vi "Append Text to Rich Text Box.vi"(8 "error in (no error)":errorcluster, 9 "Text Formatting":T1={"Font"="", "Text Color"=enum."Unchanged", "Background Color"=enum."Unchanged", "Style"=enum."Regular", "Font Size"=-1.0, "Alignment"=enum."Left"} {"Font Size" min=6.0 step=1.0}, 10 "String":string="\r\nALiX stopped on 7/2/2016 at 12:14 PM\n\r\n", 11 ".NET Refnum in":refnum<k24>) -> (0 "Error Out":errorcluster, 2 "Rtf Content":string, 3 ".NET Refnum out":refnum<k24>)   [LabVIEW 2021, in "Rich Text Box.lvlib"]
uses:
  Rich Text Box.lvlib
  System.Windows.Forms
  Text Formatting.ctl
  Text Colors.ctl
  Text Style.ctl
  Text Alignment.ctl
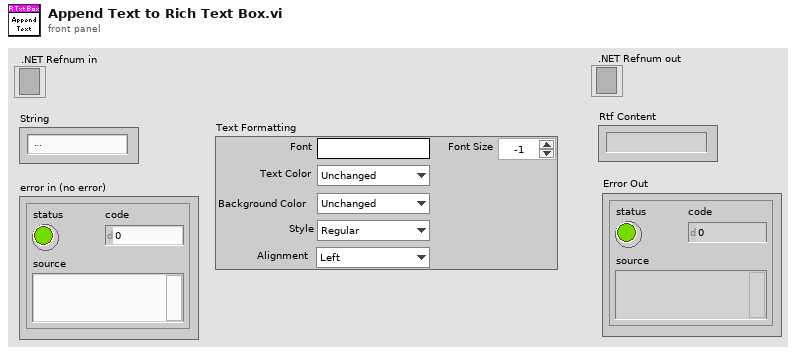
[diagram p1: front panel]
types:
  T1 = typedef "Rich Text Box.lvlib/Text Formatting.ctl" = cluster{"Font":string, "Text Color":T2, "Background Color":T2, "Style":T3, "Font Size":dbl, "Alignment":T4}
  T2 = typedef "Rich Text Box.lvlib/Text Colors.ctl" = enum16{"Unchanged", "Black", "Blue", "Cyan", "Maroon", "Gray", "Violet", "Green", "Light Green", "Orange", "Yellow", "Magenta", "Red", "White"}
  T3 = typedef "Rich Text Box.lvlib/Text Style.ctl" = enum16{"Regular", "Bold", "Italic", "Underline", "Strikeout"}
  T4 = typedef "Rich Text Box.lvlib/Text Alignment.ctl" = enum16{"Left", "Right", "Center"}
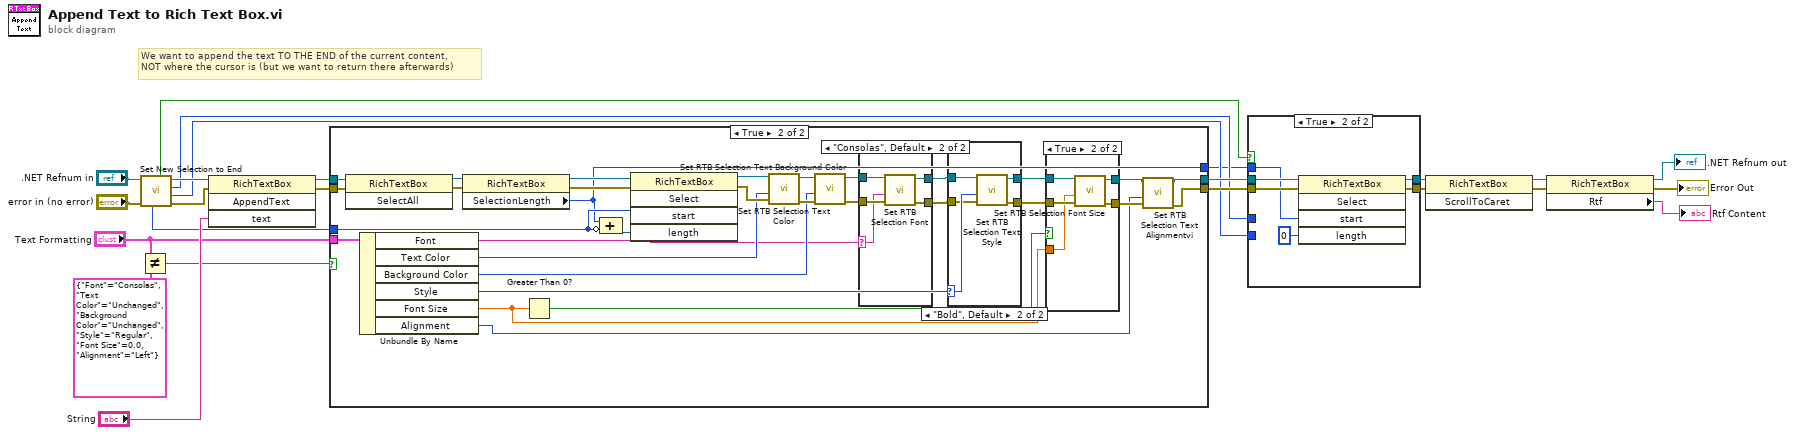
[diagram p0: block diagram]
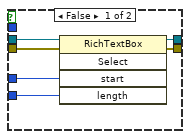
[diagram p2: hidden frame]
diagram:
  # "We want to append the text TO THE END of the current content,\nNOT where the cursor is (but we want to return there afterwards)"
  n1 = Not Equal?(x="Text Formatting", y=T1 {"Font"="Consolas", "Text Color"=enum."Unchanged", "Background Color"=enum."Unchanged", "Style"=enum."Regular", "Font Size"=0.0, "Alignment"=enum."Left"} ("Text Formatting")) -> (x != y?=w11:bool)
  n2 = call "Set New Selection to End.vi"("error in (no error)"="error in (no error)", ".NET Refnum in"=".NET Refnum in") -> ("error out"=w20:errorcluster, "Current SelectionLength"=w9:i32, "Current SelectionStart"=w10:i32, ".NET Refnum out"=w21:refnum<k24>, "Current Selection at End?"=w7:bool, "New SelectionStart: End of RTB"=w8:i32)  [unwired: 4 in]
  n3 = invoke class="RichTextBox" method="AppendText"(reference=w21, error in=w20, "text"="String") -> (reference out=w19:refnum<k24>, error out=w18:errorcluster)  [unwired: 1 in, 2 out]
  n4 = case shown="True" w11 {
    tunnel: w19 -> [w27 w58]
    tunnel: w18 -> [w26 w57]
    tunnel: w8 -> [w25 w56]
    tunnel: "Text Formatting" -> [_ w55]
    tunnel: [w26 w31] -> w13
    tunnel: [w27 w30] -> w12
    tunnel: [w25 w28] -> w6
    frame False {
    }
    frame True {
      n5 = invoke class="RichTextBox" method="SelectAll"(reference=w58, error in=w57) -> (reference out=w54:refnum<k24>, error out=w53:errorcluster)  [unwired: 1 in, 1 out]
      n6 = Unbundle By Name(w55) -> ("Font"=w38:string, "Text Color"=w47:T2, "Background Color"=w44:T2, "Style"=w43:T3, "Font Size"=w39:dbl, "Alignment"=w29:T4)
      n7 = property class="RichTextBox"(reference=w54, error in=w53) -> (reference out=w52:refnum<k24>, error out=w51:errorcluster, "SelectionLength"=w28:i32)
      n8 = Greater Than 0?(x=w39) -> (x > 0?=w42:bool)
      n9 = Compound Arithmetic op=ADD(w28, invert w56) -> (w50:i32)
      n10 = invoke class="RichTextBox" method="Select"(reference=w52, error in=w51, "start"=w56, "length"=w50) -> (reference out=w49:refnum<k24>, error out=w48:errorcluster)  [unwired: 1 in, 3 out]
      n11 = call "Set RTB Selection Text Color.vi"("Error In"=w48, "Text Color"=w47, ".NET RTB Refnum in"=w49) -> ("Error Out"=w45:errorcluster, ".NET RTB Refnum out"=w46:refnum<k24>)  [unwired: 7 in]
      n12 = call "Set RTB Selection Text Background Color.vi"("Error In"=w45, "Text Background Color"=w44, ".NET RTB Refnum in"=w46) -> ("Error Out"=w36:errorcluster, ".NET RTB Refnum out"=w37:refnum<k24>)  [unwired: 7 in]
      n13 = case shown="\"Consolas\", Default" w38 {
        selector: w38 -> [_ w61]
        tunnel: w37 -> [w60 w65]
        tunnel: w36 -> [w59 w64]
        tunnel: [w59 w63] -> w34
        tunnel: [w60 w62] -> w35
        frame "\u0000" {
        }
        frame "Consolas", Default {
          n14 = call "Set RTB Selection Font.vi"("Error In"=w64, "Font Name"=w61, ".NET RTB Refnum in"=w65) -> ("Error Out"=w63:errorcluster, ".NET RTB Refnum out"=w62:refnum<k24>)  [unwired: 7 in]
        }
      }
      n15 = case shown="\"Bold\", Default" w43 {
        selector: w43 -> [_ w78]
        tunnel: w35 -> [w74 w79]
        tunnel: w34 -> [w73 w77]
        tunnel: [w73 w76] -> w40
        tunnel: [w74 w75] -> w41
        frame "Regular" {
        }
        frame "Bold", Default {
          n16 = call "Set RTB Selection Text Style.vi"("Error In"=w77, "Style"=w78, ".NET RTB Refnum in"=w79) -> ("Error Out"=w76:errorcluster, ".NET RTB Refnum out"=w75:refnum<k24>)  [unwired: 7 in]
        }
      }
      n17 = case shown="True" w42 {
        tunnel: w41 -> [w67 w72]
        tunnel: w40 -> [w66 w71]
        tunnel: [w66 w70] -> w32
        tunnel: [w67 w69] -> w33
        tunnel: w39 -> [_ w68]
        frame False {
        }
        frame True {
          n18 = call "Set RTB Selection Font Size.vi"("Error In"=w71, "Font Size (Points)"=w68, ".NET RTB Refnum in"=w72) -> ("Error Out"=w70:errorcluster, ".NET RTB Refnum out"=w69:refnum<k24>)  [unwired: 7 in]
        }
      }
      n19 = call "Set RTB Selection Text Alignmentvi.vi"("Error In"=w32, "Text Alignment"=w29, ".NET RTB Refnum in"=w33) -> ("Error Out"=w31:errorcluster, ".NET RTB Refnum out"=w30:refnum<k24>)  [unwired: 7 in]
    }
  }
  n20 = case shown="True" w7 {
    tunnel: [w85 w91] -> w23
    tunnel: [w84 w90] -> w22
    tunnel: w13 -> [w83 w89]
    tunnel: w12 -> [w82 w88]
    tunnel: w10 -> [w81 _]
    tunnel: w9 -> [w80 _]
    tunnel: w6 -> [_ w86]
    frame False {
      n21 = invoke class="RichTextBox" method="Select"(reference=w82, error in=w83, "start"=w81, "length"=w80) -> (reference out=w85:refnum<k24>, error out=w84:errorcluster)  [unwired: 1 in, 3 out]
    }
    frame True {
      n22 = invoke class="RichTextBox" method="Select"(reference=w88, error in=w89, "start"=w86, "length"=0) -> (reference out=w91:refnum<k24>, error out=w90:errorcluster)  [unwired: 1 in, 3 out]
    }
  }
  n23 = invoke class="RichTextBox" method="ScrollToCaret"(reference=w23, error in=w22) -> (reference out=w3:refnum<k24>, error out=w5:errorcluster)  [unwired: 1 in, 1 out]
  n24 = property class="RichTextBox"(reference=w3, error in=w5) -> (reference out=→".NET Refnum out":refnum<k24>, error out=→"Error Out":errorcluster, "Rtf"=→"Rtf Content":string)
